vi "Omron TCP FINS-Release.vi"(8 "error in":errorcluster, 11 "Buffer Data":T1) -> (0 "error out":errorcluster)   [LabVIEW 2016]
uses:
  Data Def/Omron TCP FINS-Buffer Data.ctl
  Data Def/Omron TCP FINS-Command Code.ctl
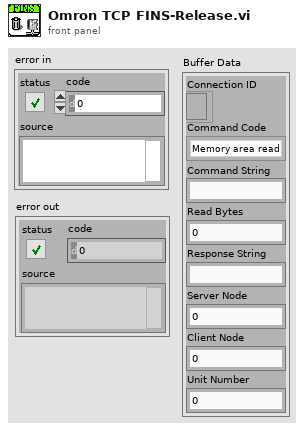
[diagram p1: front panel]
types:
  T1 = typedef "Omron TCP FINS-Buffer Data.ctl" = cluster{"Connection ID":refnum<k5>, "Command Code":T2, "Command String":string, "Read Bytes":i32, "Response String":string, "Server Node":u8, "Client Node":u8, "Unit Number":u8}
  T2 = typedef "Omron TCP FINS-Command Code.ctl" = enum16{"Memory area read", "Memory area write"}
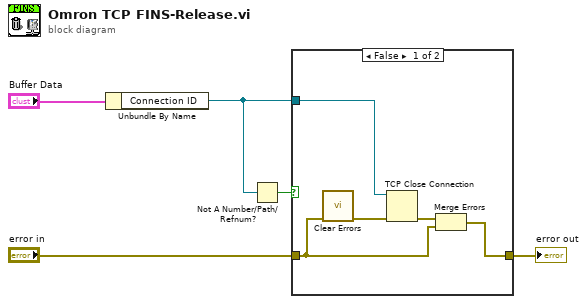
[diagram p0: block diagram]
diagram:
  n1 = Unbundle By Name("Buffer Data") -> ("Connection ID"=w3:refnum<k5>)
  n2 = Not A Number/Path/Refnum?(number/path/refnum=w3) -> (NaN/Path/Refnum?=w5:bool)
  n3 = case shown="False" w5 {
    tunnel: "error in" -> [w6 w11]
    tunnel: w3 -> [w9 _]
    tunnel: [w7 w11] -> w2
    frame False {
      n4 = call <vilib>:"Clear Errors.vi"("error in (no error)"=w6) -> ("error out"=w10:errorcluster)  [unwired: 5 in, 1 out]
      n5 = TCP Close Connection(connection ID=w9, error in (no error)=w10) -> (error out=w8:errorcluster)  [unwired: 1 in, 1 out]
      n6 = Merge Errors(w8, w6) -> (w7:errorcluster)
    }
    frame True {
    }
  }
  "error out" <- w2
